vi "AutoSteerAngle.vi"(4 "CurrentSteerAngle":dbl, 6 "CurrentDirection":dbl, 8 "Ycurrent":dbl, 9 "Xcurrent":dbl, 10 "Ywaypoint":dbl, 11 "Xwaypoint":dbl) -> (2 "NewSteerAngle":dbl)   [LabVIEW 2011]
doc: "This VI calculates steering angle from current robot position to next waypoint."
uses:
  <vilib>/addons/control/pid/pid.llb/PID (DBL).vi
  <vilib>/addons/control/pid/NI_PID_pid.lvlib
panel:
  in  "reinitialize? (F)":bool
  out "reranged":dbl
  out "SetpointCommand":dbl
  out "Waveform Chart 2":cluster{dbl, dbl}(graph)
  out "output range":cluster{"output high":dbl, "output low":dbl}={"output high"=100.0, "output low"=-100.0} {"output low" format="%.2f"; "output high" format="%.2f"}
  out "PID gains":T1={"proportional gain (Kc)"=20.0, "integral time (Ti, min)"=0.008, "derivative time (Td, min)"=0.001} {"derivative time (Td, min)" step=1e-05 format="%.5f"; "integral time (Ti, min)" step=0.0001 format="%.4f"; "proportional gain (Kc)" step=0.001 format="%.4f"}
  out "Waveform Chart":cluster{dbl, "CurrentDirection":dbl}(graph)
  out "towaypoint":dbl
  # "This Vi calculates sttering angle \nfrom current position to \nnext waypoint"
  # "0.120\n1.600\n0000"
  # "in degreees"
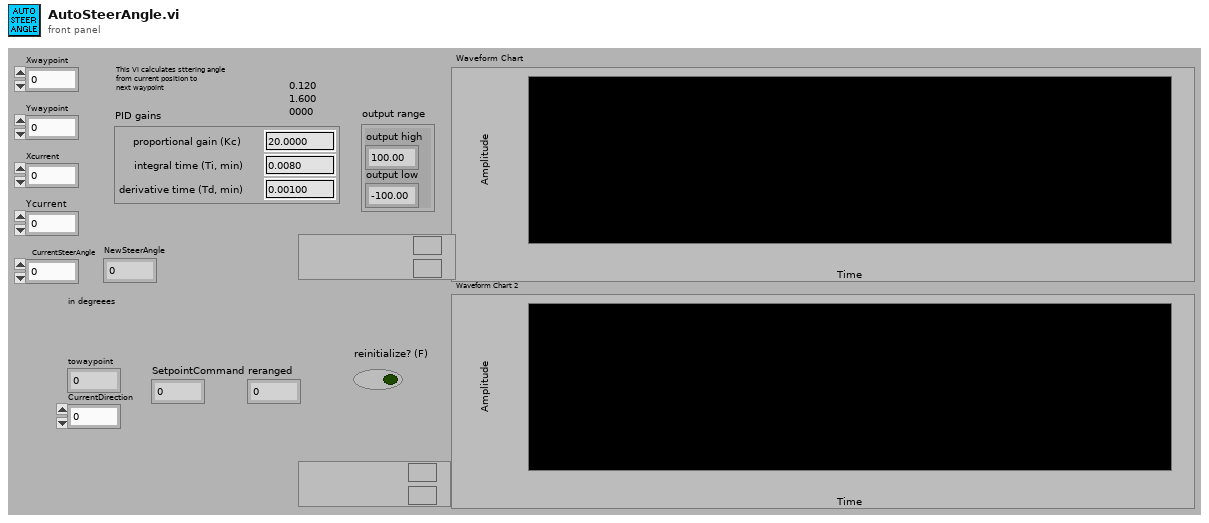
[diagram p1: front panel]
types:
  T1 = cluster{"proportional gain (Kc)":dbl, "integral time (Ti, min)":dbl, "derivative time (Td, min)":dbl}
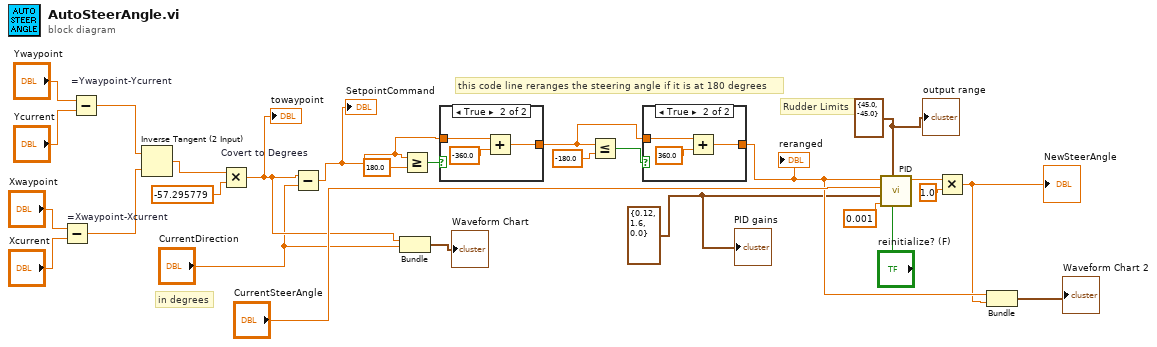
[diagram p0: block diagram]
diagram:
  w1 = T1 {"proportional gain (Kc)"=0.12, "integral time (Ti, min)"=1.6, "derivative time (Td, min)"=0.0} ("PID gains")
  w16 = cluster{"output high":dbl, "output low":dbl} {"output high"=45.0, "output low"=-45.0} ("output range")
  # "this code line reranges the steering angle if it is at 180 degrees"
  # "Rudder Limits"
  # "in degrees"
  n1 = Subtract "=Xwaypoint-Xcurrent"(x="Xwaypoint", y="Xcurrent") -> (x-y=w22:dbl)
  n2 = Subtract "=Ywaypoint-Ycurrent"(x="Ywaypoint", y="Ycurrent") -> (x-y=w23:dbl)
  n3 = Inverse Tangent (2 Input)(1:w22, 2:w23) -> (0:w20:dbl)
  n4 = Multiply "Covert to Degrees"(x=w20, y=-57.295779) -> (x*y=w8:dbl)
  "towaypoint" <- w8
  n5 = Subtract(x=w8, y="CurrentDirection") -> (x-y=w12:dbl)
  "SetpointCommand" <- w12
  n6 = Bundle(w8, "CurrentDirection"="CurrentDirection") -> (→"Waveform Chart":cluster{dbl, "CurrentDirection":dbl})  [unwired: 1 in]
  n7 = Greater Or Equal?(x=w12, y=180.0) -> (x >= y?=w13:bool)
  n8 = case shown="True" w13 {
    tunnel: w12 -> [w28 w31]
    tunnel: [w28 w29] -> w9
    frame False {
    }
    frame True {
      n9 = Add(x=w31, y=-360.0) -> (x+y=w29:dbl)
    }
  }
  n10 = Less Or Equal?(x=w9, y=-180.0) -> (x <= y?=w10:bool)
  n11 = case shown="True" w10 {
    tunnel: w9 -> [w32 w35]
    tunnel: [w32 w33] -> w5
    frame False {
    }
    frame True {
      n12 = Add(x=w35, y=360.0) -> (x+y=w33:dbl)
    }
  }
  "reranged" <- w5
  n13 = call-poly <vilib>:"PID.vi"("reinitialize? (F)"="reinitialize? (F)", "output range"=w16, "dt (s)"=0.001, "PID gains"=w1, "process variable"="CurrentSteerAngle", "setpoint"=w5) -> ("output"=w17:dbl)  [unwired: 4 in, 1 out]
  n14 = Multiply(x=w17, y=1.0) -> (x*y=w4:dbl)
  "NewSteerAngle" <- w4
  n15 = Bundle(w5, w4) -> (→"Waveform Chart 2":cluster{dbl, dbl})  [unwired: 1 in]
  "PID gains" <- w1
  "output range" <- w16
